vi "UI.vi"(8 "error in (no error)":errorcluster, 11 "View in":refnum<class "View.lvclass">) -> (0 "error out":errorcluster, 3 "View out":refnum<class "View.lvclass">)   [LabVIEW 2020, in "Container.lvlib" / "View.lvclass"]
uses:
  View.lvclass
  View.lvclass/View.ctl
panel:
  in  "Page Selector":i32(listbox)
  # "Container"
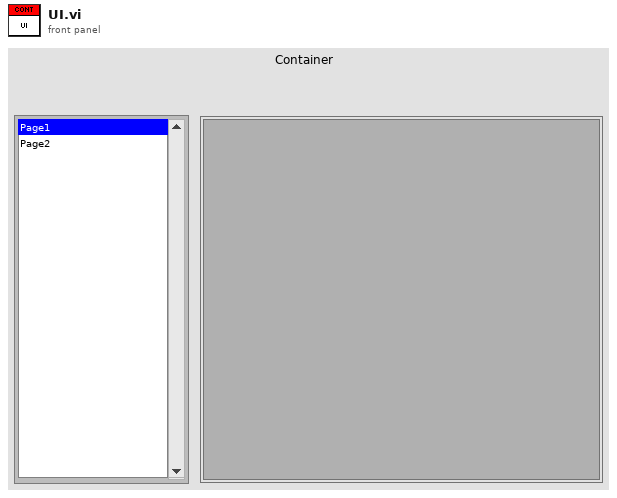
[diagram p1: front panel]
types:
  T1 = cluster{"Page Selector":refnum<vi>, "Sub Panel":refnum<vi>}
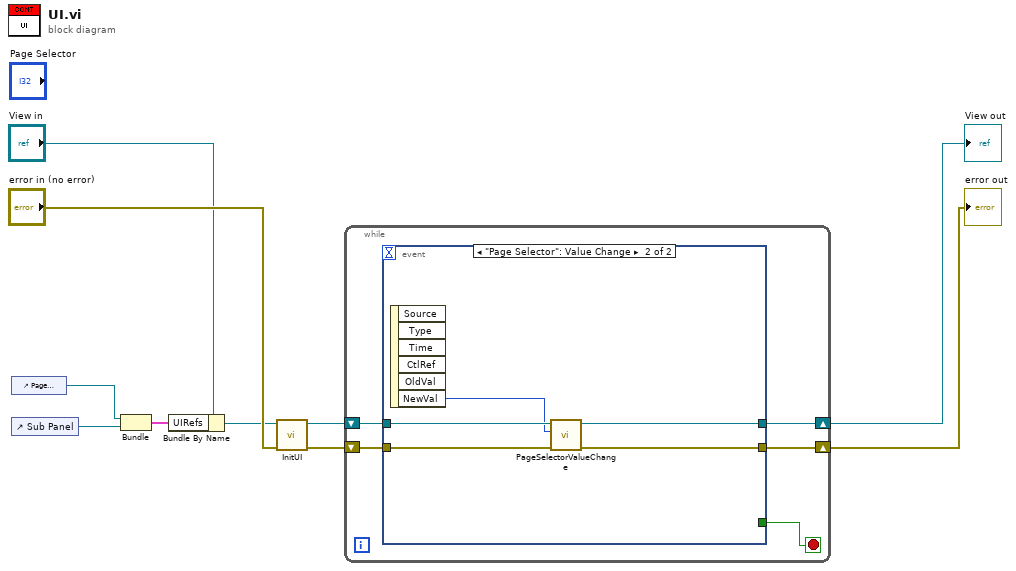
[diagram p0: block diagram]
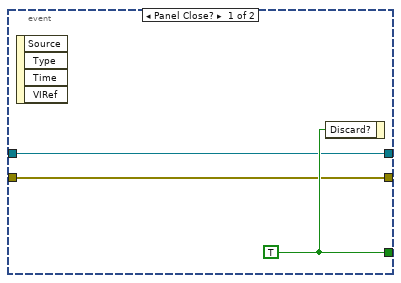
[diagram p2: hidden frame]
diagram:
  n1 = control-ref of="Page Selector"() -> (w10:refnum<vi>)
  n2 = control-ref of="Sub Panel"() -> (w8:refnum<vi>)
  n3 = Bundle("Page Selector"=w10, "Sub Panel"=w8) -> (w6:T1)  [unwired: 1 in]
  n4 = Bundle By Name(cluster="View in", "UIRefs"=w6) -> (w3:refnum<class "View.lvclass">)
  n5 = call "InitUI.vi"("error in (no error)"="error in (no error)", "View in"=w3) -> ("error out"=w2:errorcluster, "View out"=w1:refnum<class "View.lvclass">)  [unwired: 8 in]
  n6 = while {
    shift-right: [w13] -> w4
    shift-left: w2 -> [w14]
    shift-right: [w11] -> w5
    shift-left: w1 -> [w12]
    stop <- w15 stop-if-true
    n7 = event shown="[1] \"Page Selector\": Value Change" {
      selector: _ -> [_ _]
      dyn-events: _ -> [_ _]
      timeout: _ -> [_ _]
      tunnel: [w18 _] -> w15
      tunnel: w14 -> [w17 w22]
      tunnel: [w17 w20] -> w13
      tunnel: w12 -> [w16 w23]
      tunnel: [w16 w21] -> w11
      event Panel Close? {
        w18 = TRUE
        n8 = event-data() -> ()  [unwired: 1 in, 4 out]
        n9 = event-data("Discard?"=w18) -> ()  [unwired: 1 in, 1 out]
      }
      event "Page Selector": Value Change {
        n10 = event-data() -> ("NewVal"=w19:i32)  [unwired: 1 in, 5 out]
        n11 = call "PageSelectorValueChange.vi"("error in (no error)"=w22, "NewVal"=w19, "View in"=w23) -> ("error out"=w20:errorcluster, "View out"=w21:refnum<class "View.lvclass">)  [unwired: 7 in]
      }
    }
  }
  "error out" <- w4
  "View out" <- w5
